vi "水温校准.vi"() -> ()   [LabVIEW 2016, in "国弘多参数.lvlib"]
uses:
  <vilib>/Utility/config.llb/NI_LVConfig.lvlib
panel:
  in  "补偿后温度值":dbl
  out "电极温度读值":dbl
  in  "温度偏移补偿":dbl
  in  "温度电极选择":enum16{"pH电极", "电导率电极", "溶解氧电极", "浊度电极"}(ring)
  # "温度电极设定"
  # "℃"
  # "℃"
  # "℃"
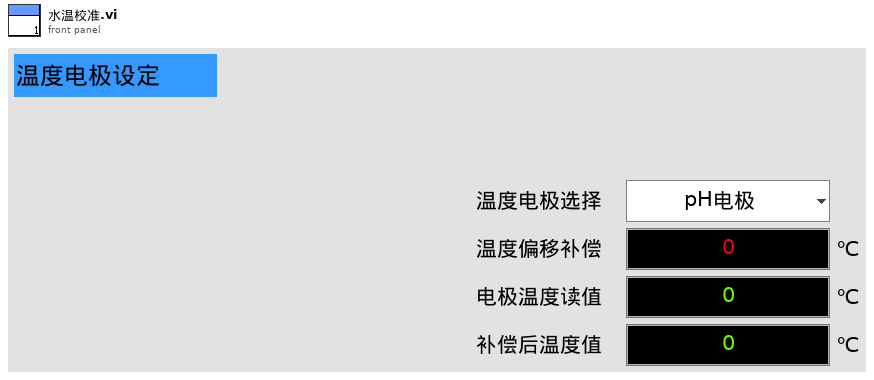
[diagram p1: front panel]
types:
  T1 = cluster{"CH":u16, "监测值":dbl, "监测信号值":dbl, "温度偏移修正值":sgl}
  T2 = typedef "NI_LVConfig.lvlib/Config Data RefNum.ctl" = refnum<k1>
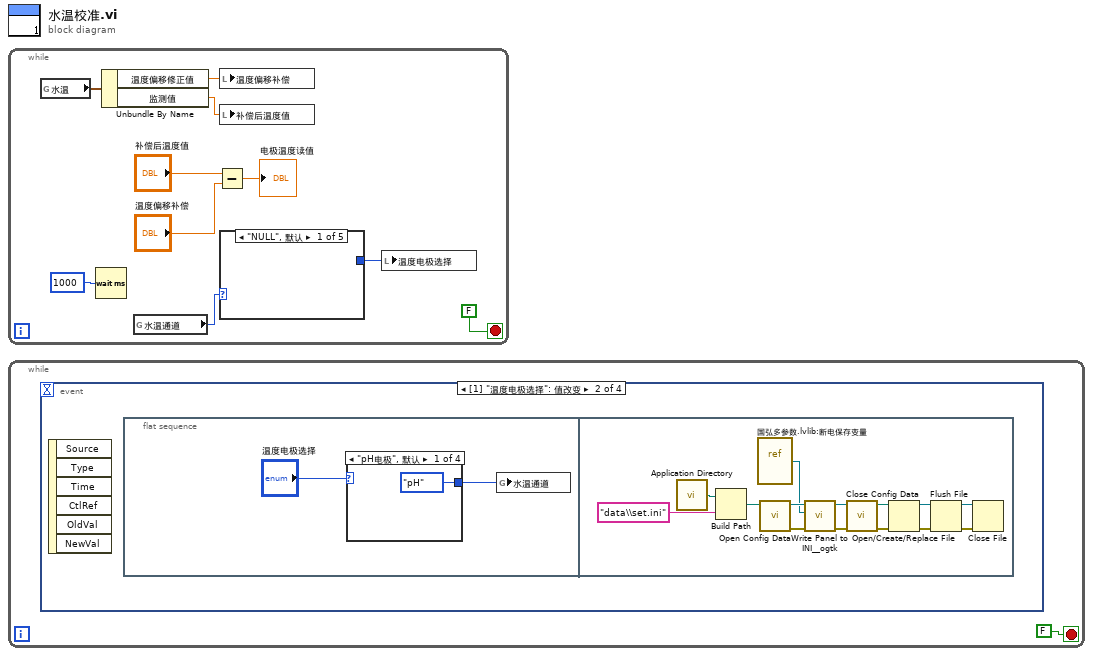
[diagram p0: block diagram]
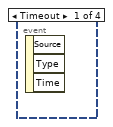
[diagram p2: hidden frame]
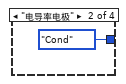
[diagram p3: hidden frame]
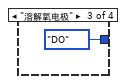
[diagram p4: hidden frame]
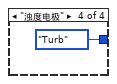
[diagram p5: hidden frame]
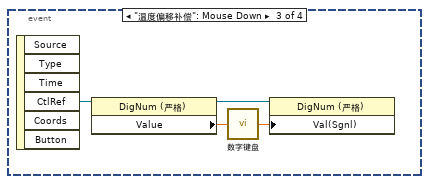
[diagram p6: hidden frame]
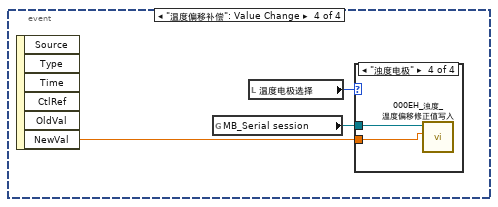
[diagram p7: hidden frame]
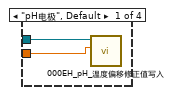
[diagram p8: hidden frame]
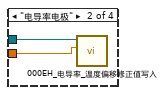
[diagram p9: hidden frame]
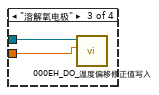
[diagram p10: hidden frame]
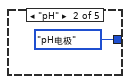
[diagram p11: hidden frame]
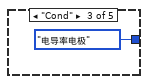
[diagram p12: hidden frame]
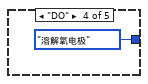
[diagram p13: hidden frame]
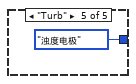
[diagram p14: hidden frame]
diagram:
  n1 = while {
    stop <- FALSE stop-if-true
    n2 = global read "过程全局变量.vi" "水温"() -> (w5:T1)
    n3 = Wait (ms)(milliseconds to wait=u32 1000 ("等待时间（毫秒）")) -> ()  [unwired: 1 out]
    n4 = Unbundle By Name(w5) -> ("温度偏移修正值"=w4:sgl, "监测值"=w3:dbl)
    n5 = global read "断电保存变量.vi" "水温通道"() -> (w2:enum16{"NULL", "pH", "Cond", "DO", "Turb"})
    n6 = Subtract(x="补偿后温度值", y="温度偏移补偿") -> (x-y=→"电极温度读值":dbl)
    n7 = local write "温度偏移补偿"(w4) -> ()
    n8 = local write "补偿后温度值"(w3) -> ()
    n9 = case shown="\"NULL\", 默认" w2 {
      tunnel: [_ enum16{"pH电极", "电导率电极", "溶解氧电极", "浊度电极"}."pH电极" ("温度电极选择") enum16{"pH电极", "电导率电极", "溶解氧电极", "浊度电极"}."电导率电极" ("温度电极选择") enum16{"pH电极", "电导率电极", "溶解氧电极", "浊度电极"}."溶解氧电极" ("温度电极选择") enum16{"pH电极", "电导率电极", "溶解氧电极", "浊度电极"}."浊度电极" ("温度电极选择")] -> w1
      frame "NULL", Default {
      }
      frame "pH" {
      }
      frame "Cond" {
      }
      frame "DO" {
      }
      frame "Turb" {
      }
    }
    n10 = local write "温度电极选择"(w1) -> ()
  }
  n11 = while {
    stop <- FALSE stop-if-true
    n12 = event shown="[1] \"温度电极选择\": 值改变" {
      selector: _ -> [_ _ _ _]
      dyn-events: _ -> [_ _ _ _]
      timeout: _ -> [_ _ _ _]
      event Timeout {
        n13 = event-data() -> ()  [unwired: 1 in, 3 out]
      }
      event "温度电极选择": Value Change {
        n14 = event-data() -> ()  [unwired: 1 in, 6 out]
        n15 = flat-sequence {
          frame #0 {
            n16 = case shown="\"pH电极\", 默认" "温度电极选择" {
              tunnel: [enum16{"NULL", "pH", "Cond", "DO", "Turb"}."pH" ("水温通道") enum16{"NULL", "pH", "Cond", "DO", "Turb"}."Cond" ("水温通道") enum16{"NULL", "pH", "Cond", "DO", "Turb"}."DO" ("水温通道") enum16{"NULL", "pH", "Cond", "DO", "Turb"}."Turb" ("水温通道")] -> w17
              frame "pH电极", Default {
              }
              frame "电导率电极" {
              }
              frame "溶解氧电极" {
              }
              frame "浊度电极" {
              }
            }
            n17 = global write "断电保存变量.vi" "水温通道"(w17) -> ()
          }
          frame #1 {
            n18 = call <vilib>:"Application Directory.vi"() -> ("Application Directory"=w31:path)
            n19 = Build Path(base path=w31, name or relative path="data\\set.ini" ("名称或相对路径")) -> (appended path=w30:path)
            n20 = vi-ref "国弘多参数.lvlib:断电保存变量.vi"() -> (w28:refnum<vi>)
            n21 = call <vilib>:"Open Config Data.vi"("configuration file path"=w30) -> ("error out"=w34:errorcluster, "refnum"=w35:T2)  [unwired: 8 in, 1 out]
            n22 = call <userlib>:"Write Panel to INI__ogtk.vi"("error in (no error)"=w34, "VI ref"=w28, "refnum"=w35) -> ("error out"=w32:errorcluster, "refnum out"=w33:T2)  [unwired: 7 in]
            n23 = call <vilib>:"Close Config Data.vi"("error in (no error)"=w32, "refnum"=w33) -> ("error out"=w24:errorcluster, "file path"=w25:path)  [unwired: 8 in]
            n24 = Open/Create/Replace File(file path (use dialog)=w25, error in=w24) -> (refnum out=w26:refnum<file>, error out=w27:errorcluster)  [unwired: 4 in, 1 out]
            n25 = Flush File(refnum=w26, error in=w27) -> (refnum out=w22:refnum<file>, error out=w23:errorcluster)
            n26 = Close File(refnum=w22, error in=w23) -> ()  [unwired: 2 out]
          }
        }
      }
      event "温度偏移补偿": Mouse Down {
        n27 = event-data() -> ("CtlRef"=w39:refnum<vi>)  [unwired: 1 in, 5 out]
        n28 = property class="DigNum (严格)"(reference=w39) -> (reference out=w36:refnum<vi>, "Value"=w38:dbl)  [unwired: 1 in, 1 out]
        n29 = call "数字键盘.vi"("OldNumber"=w38) -> ("NewNumber"=w37:sgl)
        n30 = property class="DigNum (严格)"(reference=w36, "Val(Sgnl)"=w37) -> ()  [unwired: 1 in, 2 out]
      }
      event "温度偏移补偿": Value Change {
        n31 = event-data() -> ("NewVal"=w41:dbl)  [unwired: 1 in, 5 out]
        n32 = global read "过程全局变量.vi" "MB_Serial session"() -> (w40:refnum<class "MB_Master_Serial.lvclass">)
        n33 = local read "温度电极选择"() -> (w42:enum16{"pH电极", "电导率电极", "溶解氧电极", "浊度电极"})
        n34 = case shown="\"浊度电极\"" w42 {
          tunnel: w41 -> [w44 w46 w48 w50]
          tunnel: w40 -> [w43 w45 w47 w49]
          frame "pH电极", Default {
            n35 = call "000EH_pH_温度偏移修正值写入.vi"("数值"=w44, "MB_Serial session in"=w43) -> ()  [unwired: 8 in, 2 out]
          }
          frame "电导率电极" {
            n36 = call "000EH_电导率_温度偏移修正值写入.vi"("数值"=w46, "MB_Serial session in"=w45) -> ()  [unwired: 8 in, 2 out]
          }
          frame "溶解氧电极" {
            n37 = call "000EH_DO_温度偏移修正值写入.vi"("数值"=w48, "MB_Serial session in"=w47) -> ()  [unwired: 8 in, 2 out]
          }
          frame "浊度电极" {
            n38 = call "000EH_浊度_温度偏移修正值写入.vi"("数值"=w50, "MB_Serial session in"=w49) -> ()  [unwired: 8 in, 2 out]
          }
        }
      }
    }
  }
